vi "Part based Initialization_DL.vi"(8 "error in (no error)":errorcluster, 10 "Part Info":T1, 11 "DataLogger in":refnum<class "DataLogger.lvclass">) -> (0 "error out":errorcluster, 3 "DataLogger out":refnum<class "DataLogger.lvclass">)   [LabVIEW 2019, in "DataLogger.lvclass"]
uses:
  DataLogger.lvclass
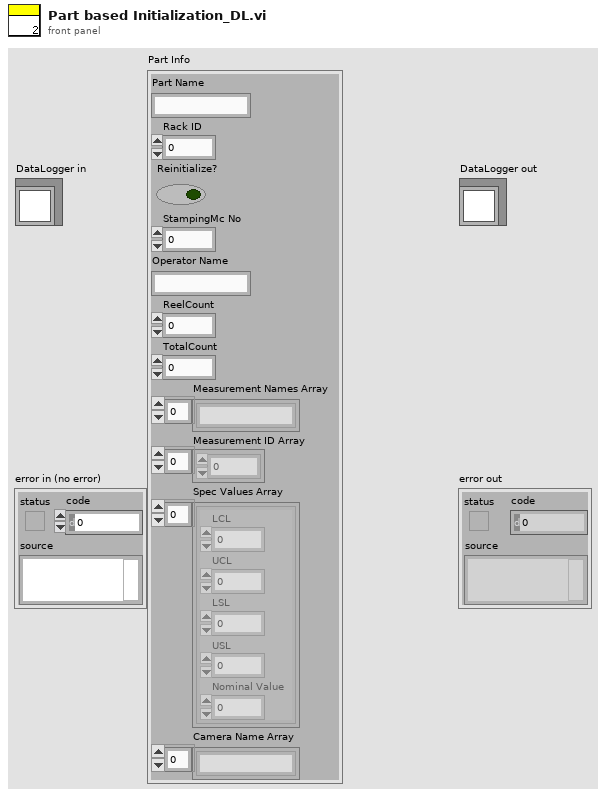
[diagram p1: front panel]
types:
  T1 = cluster{"Part Name":string, "Rack ID":u8, "Reinitialize?":bool, "StampingMc No":u64, "Operator Name":string, "ReelCount":u64, "TotalCount":u64, "Measurement Names Array":string[], "Measurement ID Array":u16[], "Spec Values Array":cluster{"LCL":dbl, "UCL":dbl, "LSL":dbl, "USL":dbl, "Nominal Value":dbl}[], "Camera Name Array":string[]}
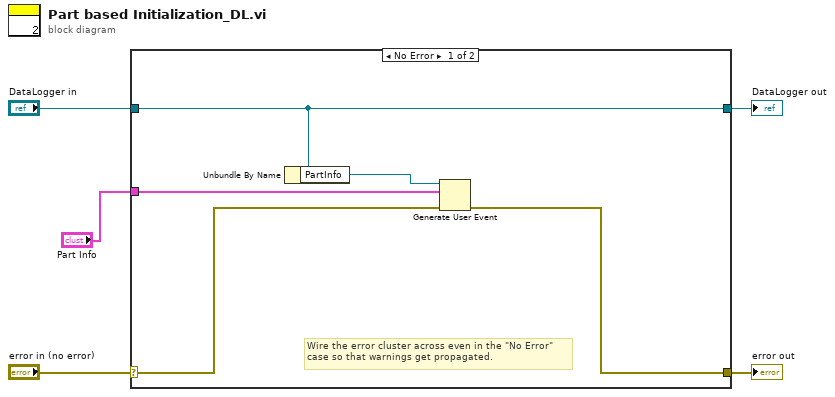
[diagram p0: block diagram]
diagram:
  n1 = case shown="No Error" "error in (no error)" {
    selector: "error in (no error)" -> [w7 w12]
    tunnel: [w6 w12] -> w4
    tunnel: [w10 w11] -> w2
    tunnel: "DataLogger in" -> [w10 w11]
    tunnel: "Part Info" -> [w8 _]
    frame No Error {
      # "Wire the error cluster across even in the \"No Error\"\ncase so that warnings get propagated."
      n2 = Unbundle By Name(w10) -> ("PartInfo"=w9:refnum<user-event>)
      n3 = Generate User Event(user event=w9, event data cluster=w8, error in=w7) -> (error out=w6:errorcluster)  [unwired: 1 in, 1 out]
    }
    frame Error {
    }
  }
  "error out" <- w4
  "DataLogger out" <- w2
